vi "SendCMD.vi"(8 "error in (no error)":errorcluster, 10 "Vision_Modes":T1=enum."ResetCamera", 11 "Camera Port In":refnum<visa-resource-name>) -> (0 "error out":errorcluster, 3 "Camera Port Out":refnum<visa-resource-name>)   [LabVIEW 2017, in "VisionHW.lvlib"]
uses:
  VisionHW.lvlib
  TypeDefs/ENUM_Vision_Commands.ctl
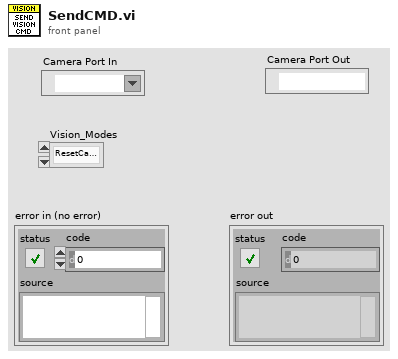
[diagram p1: front panel]
types:
  T1 = typedef "ENUM_Vision_Commands.ctl" = enum16{"Init", "NoOp", "ResetCamera", "VideoOn", "VideoOff", "CubeDetection", "RoadNavigation"}
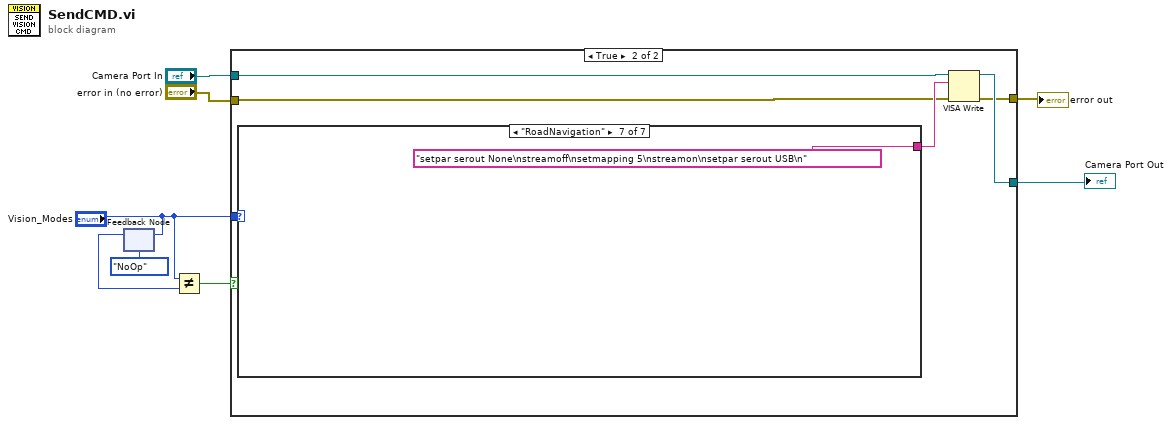
[diagram p0: block diagram]
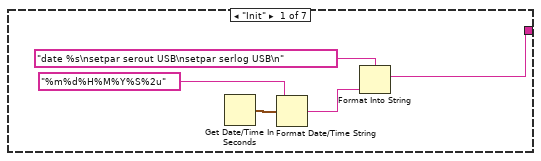
[diagram p3: hidden frame]
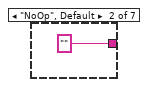
[diagram p4: hidden frame]
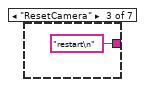
[diagram p5: hidden frame]
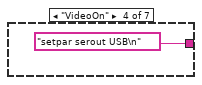
[diagram p6: hidden frame]
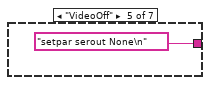
[diagram p7: hidden frame]
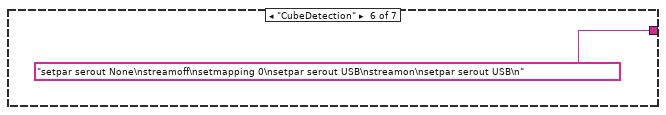
[diagram p8: hidden frame]
diagram:
  n1 = feedback-in #1("Vision_Modes") -> ()
  n2 = feedback #1(ENUM_Vision_Commands."NoOp" ("Vision_Modes")) -> (w5:T1)
  n3 = Not Equal?(x="Vision_Modes", y=w5) -> (x != y?=w3:bool)
  n4 = case shown="True" w3 {
    tunnel: "Vision_Modes" -> [_ w16]
    tunnel: "Camera Port In" -> [w10 w14]
    tunnel: [w10 w13] -> w7
    tunnel: "error in (no error)" -> [w9 w12]
    tunnel: [w9 w11] -> w1
    frame False {
    }
    frame True {
      n5 = case shown="\"RoadNavigation\"" w16 {
        tunnel: [w17 "" "restart\n" "setpar serout USB\n" "setpar serout None\n" "setpar serout None\nstreamoff\nsetmapping 0\nsetpar serout USB\nstreamon\nsetpar serout USB\n" "setpar serout None\nstreamoff\nsetmapping 5\nstreamon\nsetpar serout USB\n"] -> w15
        frame "Init" {
          n6 = Get Date/Time In Seconds() -> (seconds since 1Jan1904=w21:timestamp)
          n7 = Format Date/Time String(time format string (%c)="%m%d%H%M%Y%S%2u", seconds (now)=w21) -> (date/time string=w18:string)  [unwired: 1 in]
          n8 = Format Into String(format string="date %s\nsetpar serout USB\nsetpar serlog USB\n" ("write buffer"), w18) -> (resulting string=w17:string)  [unwired: 2 in, 1 out]
        }
        frame "NoOp", Default {
        }
        frame "ResetCamera" {
        }
        frame "VideoOn" {
        }
        frame "VideoOff" {
        }
        frame "CubeDetection" {
        }
        frame "RoadNavigation" {
        }
      }
      n9 = VISA Write(VISA resource name=w14, write buffer=w15, error in (no error)=w12) -> (VISA resource name out=w13:refnum<visa-resource-name>, error out=w11:errorcluster)  [unwired: 1 out]
    }
  }
  "error out" <- w1
  "Camera Port Out" <- w7
